vi "Log Motor FB.vi"(8 "error in":errorcluster, 10 "MFB":T1, 11 "tdms file in":refnum<k34>) -> (0 "error out":errorcluster, 3 "tdms file in":refnum<k34>)   [LabVIEW 2022 SP3]
uses:
  <vilib>/Waveform/WDTOps.llb/WDT Get Waveform Time Array DBL.vi
panel:
  out "x":u32
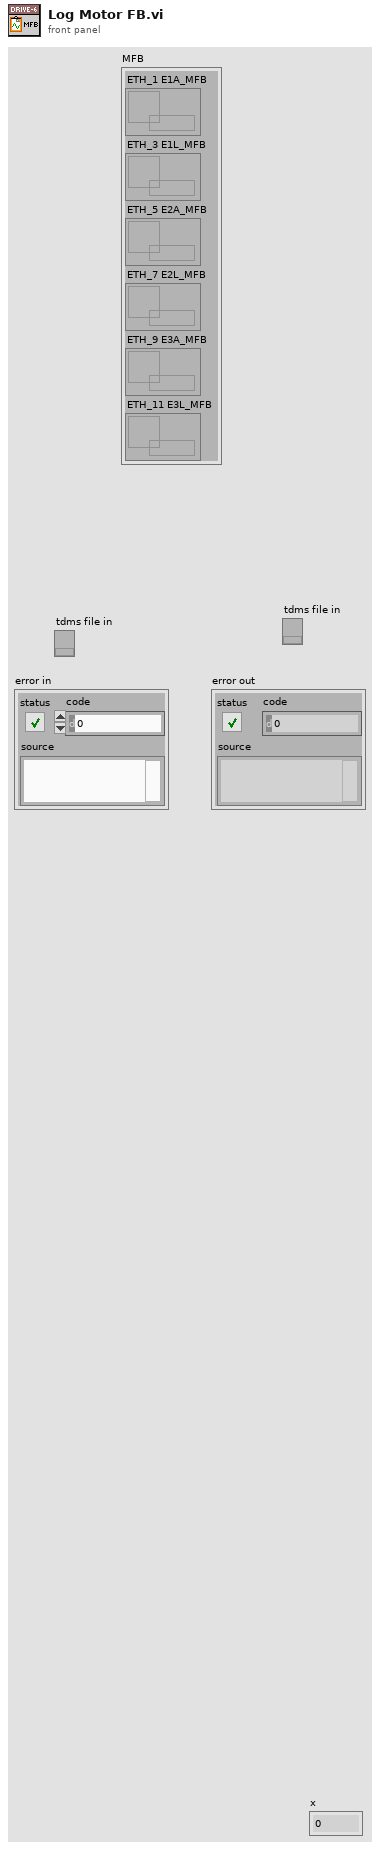
[diagram p1: front panel]
types:
  T1 = cluster{"ETH_1 E1A_MFB":refnum<queue>, "ETH_3 E1L_MFB":refnum<queue>, "ETH_5 E2A_MFB":refnum<queue>, "ETH_7 E2L_MFB":refnum<queue>, "ETH_9 E3A_MFB":refnum<queue>, "ETH_11 E3L_MFB":refnum<queue>}
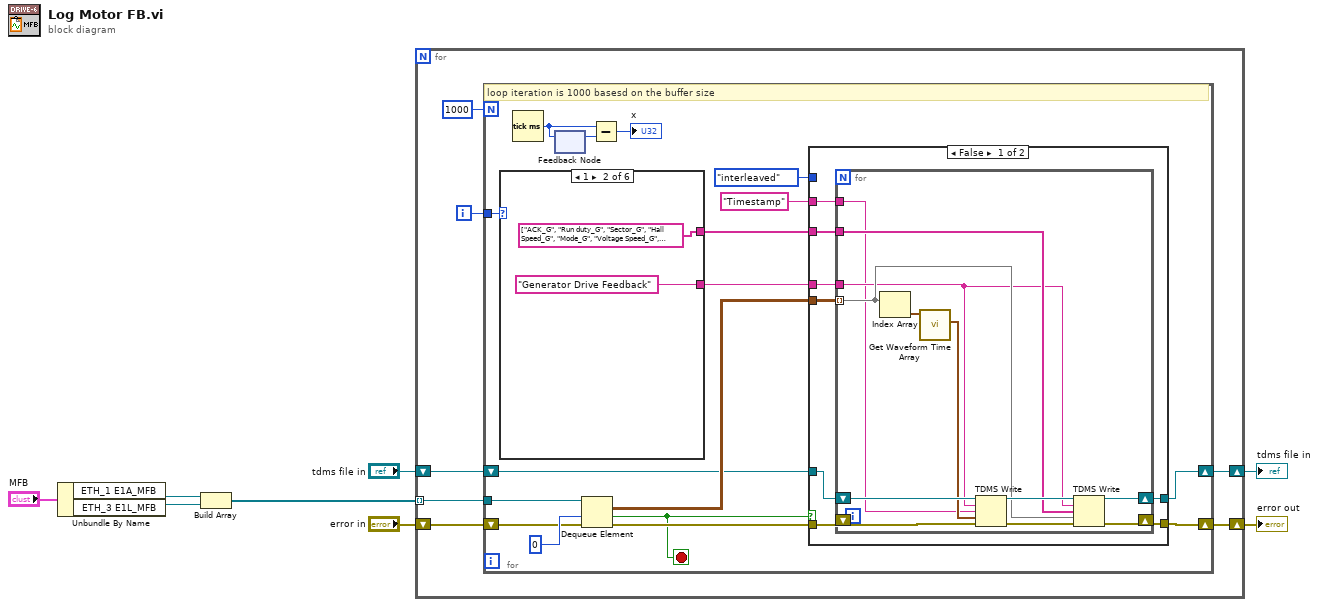
[diagram p0: block diagram]
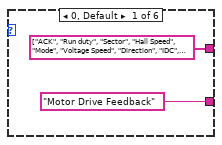
[diagram p3: hidden frame]
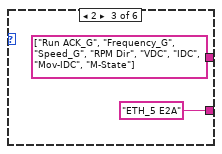
[diagram p4: hidden frame]
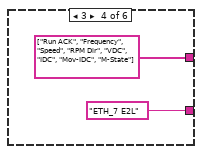
[diagram p5: hidden frame]
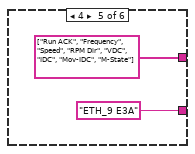
[diagram p6: hidden frame]
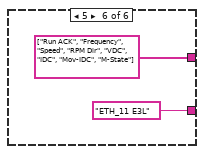
[diagram p7: hidden frame]
diagram:
  n1 = Unbundle By Name("MFB") -> ("ETH_1 E1A_MFB"=w5:refnum<queue>, "ETH_3 E1L_MFB"=w4:refnum<queue>)
  n2 = Build Array(w5, w4) -> (w3:refnum<queue>[])
  n3 = for {
    tunnel: w3 -> [w14] mode=indexing
    shift-right: [w12] -> w2
    shift-left: "tdms file in" -> [w15]
    shift-right: [w10] -> w1
    shift-left: "error in" -> [w11]
    i -> [w9]
    n4 = for {
      N: 1000 -> [_]
      tunnel: w14 -> [w30]
      shift-right: [w22] -> w12
      shift-left: w15 -> [w20]
      shift-right: [w21] -> w10
      shift-left: w11 -> [w29]
      tunnel: w9 -> [w32]
      stop <- w18 stop-if-true
      # "loop iteration is 1000 basesd on the buffer size"
      n5 = case shown="1" w32 {
        tunnel: [string[] ["ACK", "Run duty", "Sector", "Hall Speed", "Mode", "Voltage Speed", "Direction", "IDC", "Movable Average", "VDC"] ("channel name(s) in (Untitled)") string[] ["ACK_G", "Run duty_G", "Sector_G", "Hall Speed_G", "Mode_G", "Voltage Speed_G", "Direction_G", "IDC_G", "Movable Average_G", "VDC_G"] ("channel name(s) in (Untitled)") string[] ["Run ACK_G", "Frequency_G", "Speed_G", "RPM Dir", "VDC", "IDC", "Mov-IDC", "M-State"] ("appended array") string[] ["Run ACK", "Frequency", "Speed", "RPM Dir", "VDC", "IDC", "Mov-IDC", "M-State"] ("appended array") string[] ["Run ACK", "Frequency", "Speed", "RPM Dir", "VDC", "IDC", "Mov-IDC", "M-State"] ("appended array") string[] ["Run ACK", "Frequency", "Speed", "RPM Dir", "VDC", "IDC", "Mov-IDC", "M-State"] ("appended array")] -> w23
        tunnel: ["Motor Drive Feedback" ("group name in (Untitled)") "Generator Drive Feedback" ("group name in (Untitled)") "ETH_5 E2A" ("group name in (Untitled)") "ETH_7 E2L" ("group name in (Untitled)") "ETH_9 E3A" ("group name in (Untitled)") "ETH_11 E3L" ("group name in (Untitled)")] -> w24
        frame 0, Default {
        }
        frame 1 {
        }
        frame 2 {
        }
        frame 3 {
        }
        frame 4 {
        }
        frame 5 {
        }
      }
      n6 = Tick Count (ms)() -> (millisecond timer value=w27:u32)
      n7 = feedback #1() -> (w28:u32)  [unwired: 1 in]
      n8 = feedback-in #1(w27) -> ()
      n9 = Dequeue Element(queue=w30, timeout in ms (-1)=0, error in (no error)=w29) -> (element=w25:waveform(dbl)[][], timed out?=w18:bool, error out=w19:errorcluster)  [unwired: 1 out]
      n10 = Subtract(x=w27, y=w28) -> (x-y=→"x":u32)
      n11 = case shown="False" w18 {
        tunnel: [w40 w53] -> w21
        tunnel: [w39 w54] -> w22
        tunnel: w24 -> [w35 _]
        tunnel: "Timestamp" -> [w33 _]
        tunnel: w23 -> [w34 _]
        tunnel: w25 -> [w36 _]
        tunnel: enum16{"decimated", "interleaved"}."interleaved" ("data layout (0:decimated)") -> [_ _]
        tunnel: w20 -> [w37 w54]
        tunnel: w19 -> [w38 w53]
        frame False {
          n12 = for {
            shift-right: [w51] -> w40
            shift-left: w38 -> [w48]
            shift-right: [w49] -> w39
            shift-left: w37 -> [w47]
            tunnel: w36 -> [w44] mode=indexing
            tunnel: w35 -> [w42]
            tunnel: w34 -> [w43]
            tunnel: w33 -> [w41]
            n13 = Index Array(array=w44) -> (element=w46:waveform(dbl))  [unwired: 1 in]
            n14 = call-poly <vilib>:"Get Waveform Time Array.vi"("waveform in"=w46) -> ("X array"=w45:timestamp[])  [unwired: 9 in, 1 out]
            n15 = TDMS Write(0:w47, 5:w42, 7:w41, 9:w45, 11:w48) -> (4:w50:refnum<k34>, 15:w52:errorcluster)  [unwired: 1 in, 2 out]
            n16 = TDMS Write(0:w50, 5:w42, 7:w43, 9:w44, 11:w52) -> (4:w49:refnum<k34>, 15:w51:errorcluster)  [unwired: 1 in, 2 out]
          }
        }
        frame True {
        }
      }
    }
  }
  "tdms file in" <- w2
  "error out" <- w1
